vi "Write selected.vi"(8 "error in (no error)":errorcluster, 10 "selected":bool, 11 "GObject in":refnum<class "GObject.lvclass">) -> (0 "error out":errorcluster, 3 "GObject out":refnum<class "GObject.lvclass">)   [LabVIEW 2023, in "TLC_Scripto.lvlib" / "GObject.lvclass"]
uses:
  GObject.lvclass
  GObject.lvclass/GObject.ctl
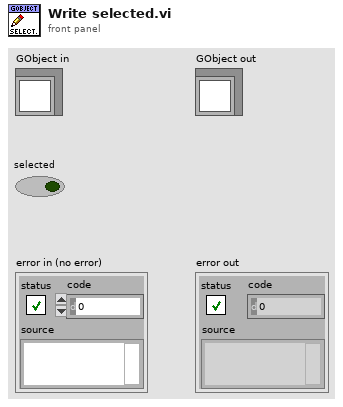
[diagram p1: front panel]
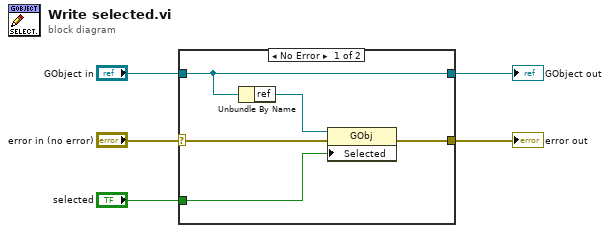
[diagram p0: block diagram]
diagram:
  n1 = case shown="No Error" "error in (no error)" {
    selector: "error in (no error)" -> [w7 w12]
    tunnel: [w6 w12] -> w4
    tunnel: [w10 w11] -> w2
    tunnel: "GObject in" -> [w10 w11]
    tunnel: "selected" -> [w8 _]
    frame No Error {
      n2 = Unbundle By Name(w10) -> ("ref"=w9:refnum<vi>)
      n3 = property class="GObj"(reference=w9, error in=w7, "Selected"=w8) -> (error out=w6:errorcluster)  [unwired: 1 out]
    }
    frame Error {
    }
  }
  "error out" <- w4
  "GObject out" <- w2
